vi "Read Measurement (Burst Average Power).vi"(0 "VISA resource name":refnum<visa-resource-name>, 11 "error in (no error)":errorcluster) -> (4 "VISA resource name out":refnum<visa-resource-name>, 6 "Burst Average Power":dbl, 15 "error out":errorcluster)   [LabVIEW 2020, in "Anritsu Signal Analyzer Series.lvlib"]
doc: "Reads Burst Average Power measurement data"
uses:
  Anritsu Signal Analyzer Series.lvlib
panel:
  # "dBm"
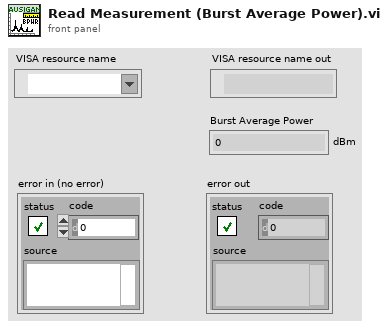
[diagram p1: front panel]
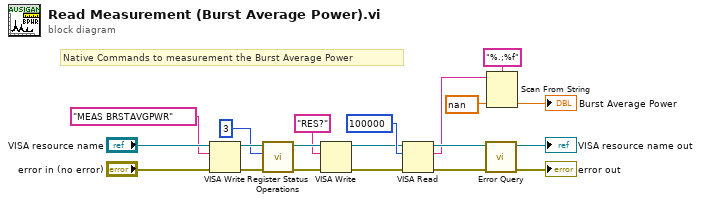
[diagram p0: block diagram]
diagram:
  # "Native Commands to measurement the Burst Average Power"
  n1 = VISA Write(VISA resource name="VISA resource name", write buffer="MEAS BRSTAVGPWR" ("_CommandSet"), error in (no error)="error in (no error)") -> (VISA resource name out=w13:refnum<visa-resource-name>, error out=w12:errorcluster)  [unwired: 1 out]
  n2 = call "Register Status Operations.vi"("error in (no error)"=w12, "Register (0:*SRE)"=3, "VISA resource name"=w13) -> ("error out"=w10:errorcluster, "VISA resource name out"=w11:refnum<visa-resource-name>)  [unwired: 6 in, 1 out]
  n3 = VISA Write(VISA resource name=w11, write buffer="RES?" ("_Command"), error in (no error)=w10) -> (VISA resource name out=w8:refnum<visa-resource-name>, error out=w7:errorcluster)  [unwired: 1 out]
  n4 = VISA Read(VISA resource name=w8, byte count=u32 100000 ("byte count (0)"), error in (no error)=w7) -> (VISA resource name out=w5:refnum<visa-resource-name>, read buffer=w2:string, error out=w6:errorcluster)  [unwired: 1 out]
  n5 = call "Error Query.vi"("error in (no error)"=w6, "VISA resource name"=w5) -> ("error out"=→"error out":errorcluster, "VISA resource name out"=→"VISA resource name out":refnum<visa-resource-name>)  [unwired: 6 in, 2 out]
  n6 = Scan From String(format string="%.;%f" ("Format String"), input string=w2, default 1=nan ("_Default")) -> (output 1=→"Burst Average Power":dbl)  [unwired: 2 in, 3 out]
